vi "Adj Controls Pos.vi"(0 "Decoration Ref Array":refnum<vi>[](array[refnum]), 2 "Panel Bounds":T1, 11 "Control Ref Array":refnum<vi>[](array[refnum])) -> ()   [LabVIEW 2021]
uses:
  <vilib>/Utility/miscctls.llb/LVRectTypeDef.ctl
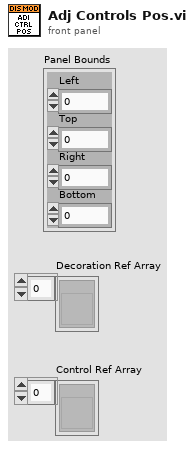
[diagram p1: front panel]
types:
  T1 = typedef "LVRectTypeDef.ctl" = cluster{"Left":i16, "Top":i16, "Right":i16, "Bottom":i16}
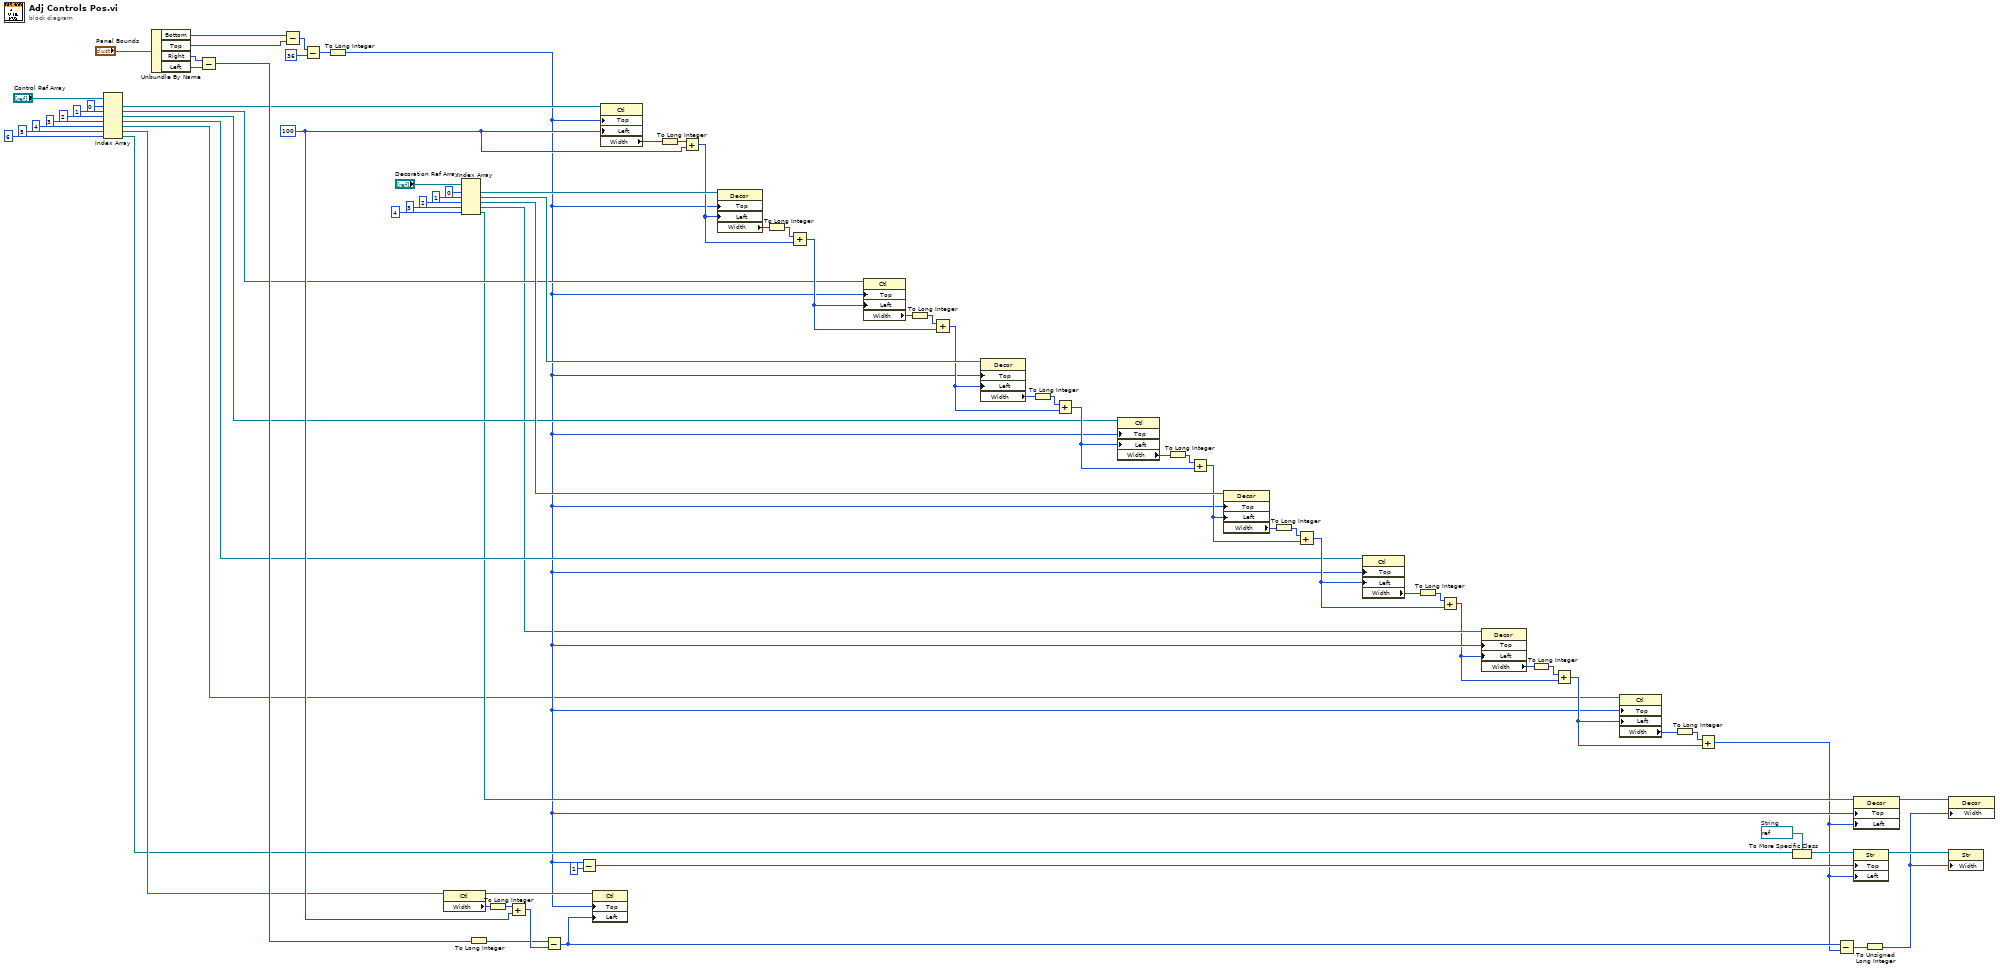
[diagram p0: block diagram]
diagram:
  w15 = refnum<vi> refnum  # String
  w70 = 100 ("Position:Left")
  n1 = Index Array(array="Control Ref Array", index #1=0 ("index"), index #2=1 ("index"), index #3=2 ("index"), index #4=3 ("index"), index #5=4 ("index"), index #6=5 ("index"), index #7=6 ("index")) -> (element #1=w20:refnum<vi>, element #2=w19:refnum<vi>, element #3=w18:refnum<vi>, element #4=w16:refnum<vi>, element #5=w3:refnum<vi>, element #6=w17:refnum<vi>, element #7=w14:refnum<vi>)
  n2 = Unbundle By Name("Panel Bounds") -> ("Bottom"=w75:i16, "Top"=w74:i16, "Right"=w73:i16, "Left"=w72:i16)
  n3 = Subtract(x=w73, y=w72) -> (x-y=w69:i16)
  n4 = Subtract(x=w75, y=w74) -> (x-y=w78:i16)
  n5 = Subtract(x=w78, y=i16 36) -> (x-y=w71:i16)
  n6 = To Long Integer(number=w71) -> (32bit integer=w5:i32)
  n7 = property class="Ctl"(reference=w17) -> (reference out=w55:refnum<vi>, "Width"=w54:u32)  [unwired: 1 in, 1 out]
  n8 = Index Array(array="Decoration Ref Array", index #1=0 ("index"), index #2=1 ("index"), index #3=2 ("index"), index #4=3 ("index"), index #5=4 ("index")) -> (element #1=w68:refnum<vi>, element #2=w43:refnum<vi>, element #3=w37:refnum<vi>, element #4=w4:refnum<vi>, element #5=w11:refnum<vi>)
  n9 = To Long Integer(number=w69) -> (32bit integer=w51:i32)
  n10 = To Long Integer(number=w54) -> (32bit integer=w53:i32)
  n11 = Add(x=w53, y=w70) -> (x+y=w52:i32)
  n12 = Subtract(x=w51, y=w52) -> (x-y=w48:i32)
  n13 = Subtract(x=w5, y=1) -> (x-y=w65:i32)
  n14 = property class="Ctl"(reference=w55, "Top"=w5, "Left"=w48) -> ()  [unwired: 1 in, 2 out]
  n15 = property class="Ctl"(reference=w20, "Top"=w5, "Left"=w70) -> ("Width"=w63:u32)  [unwired: 1 in, 2 out]
  n16 = To Long Integer(number=w63) -> (32bit integer=w62:i32)
  n17 = Add(x=w62, y=w70) -> (x+y=w57:i32)
  n18 = property class="Decor"(reference=w68, "Top"=w5, "Left"=w57) -> ("Width"=w61:u32)  [unwired: 1 in, 2 out]
  n19 = To Long Integer(number=w61) -> (32bit integer=w60:i32)
  n20 = Add(x=w60, y=w57) -> (x+y=w56:i32)
  n21 = property class="Ctl"(reference=w19, "Top"=w5, "Left"=w56) -> ("Width"=w58:u32)  [unwired: 1 in, 2 out]
  n22 = To Long Integer(number=w58) -> (32bit integer=w59:i32)
  n23 = Add(x=w59, y=w56) -> (x+y=w40:i32)
  n24 = property class="Decor"(reference=w43, "Top"=w5, "Left"=w40) -> ("Width"=w41:u32)  [unwired: 1 in, 2 out]
  n25 = To Long Integer(number=w41) -> (32bit integer=w42:i32)
  n26 = Add(x=w42, y=w40) -> (x+y=w36:i32)
  n27 = property class="Ctl"(reference=w18, "Top"=w5, "Left"=w36) -> ("Width"=w38:u32)  [unwired: 1 in, 2 out]
  n28 = To Long Integer(number=w38) -> (32bit integer=w39:i32)
  n29 = Add(x=w39, y=w36) -> (x+y=w33:i32)
  n30 = property class="Decor"(reference=w37, "Top"=w5, "Left"=w33) -> ("Width"=w34:u32)  [unwired: 1 in, 2 out]
  n31 = To Long Integer(number=w34) -> (32bit integer=w35:i32)
  n32 = Add(x=w35, y=w33) -> (x+y=w30:i32)
  n33 = property class="Ctl"(reference=w16, "Top"=w5, "Left"=w30) -> ("Width"=w31:u32)  [unwired: 1 in, 2 out]
  n34 = To Long Integer(number=w31) -> (32bit integer=w32:i32)
  n35 = Add(x=w32, y=w30) -> (x+y=w2:i32)
  n36 = property class="Decor"(reference=w4, "Top"=w5, "Left"=w2) -> ("Width"=w7:u32)  [unwired: 1 in, 2 out]
  n37 = To Long Integer(number=w7) -> (32bit integer=w6:i32)
  n38 = Add(x=w6, y=w2) -> (x+y=w10:i32)
  n39 = property class="Ctl"(reference=w3, "Top"=w5, "Left"=w10) -> ("Width"=w9:u32)  [unwired: 1 in, 2 out]
  n40 = To Long Integer(number=w9) -> (32bit integer=w8:i32)
  n41 = Add(x=w8, y=w10) -> (x+y=w1:i32)
  n42 = To More Specific Class(target class=w15, reference=w14) -> (specific class reference=w13:refnum<vi>)  [unwired: 1 in, 1 out]
  n43 = Subtract(x=w48, y=w1) -> (x-y=w47:i32)
  n44 = property class="Decor"(reference=w11, "Top"=w5, "Left"=w1) -> (reference out=w50:refnum<vi>)  [unwired: 1 in, 1 out]
  n45 = property class="Str"(reference=w13, "Top"=w65, "Left"=w1) -> (reference out=w49:refnum<vi>)  [unwired: 1 in, 1 out]
  n46 = To Unsigned Long Integer(number=w47) -> (unsigned 32bit integer=w46:u32)
  n47 = property class="Decor"(reference=w50, "Width"=w46) -> ()  [unwired: 1 in, 2 out]
  n48 = property class="Str"(reference=w49, "Width"=w46) -> ()  [unwired: 1 in, 2 out]
